vi "air formulas (SubVI).vi"(6 "Airflow Offset":dbl, 9 "Air Pressure Offset":dbl, 10 "Numeric in":u16, 11 "Numeric 4":u16) -> (2 "Numeric out":dbl, 3 "Numeric 3":dbl)   [LabVIEW 2016]
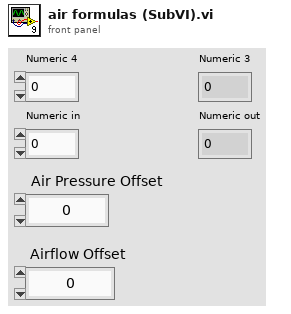
[diagram p1: front panel]
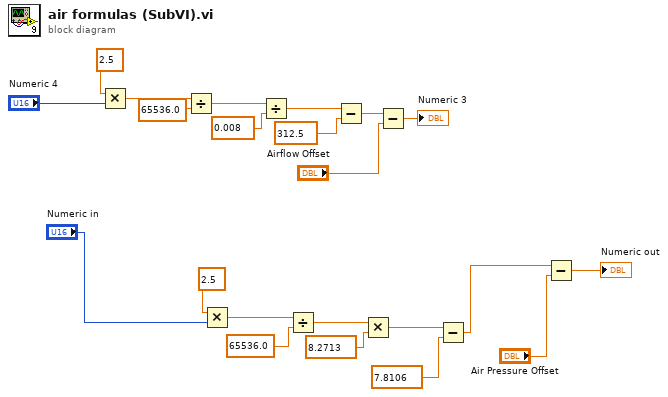
[diagram p0: block diagram]
diagram:
  n1 = Multiply(x=2.5, y="Numeric 4") -> (x*y=w12:dbl)
  n2 = Divide(x=w12, y=65536.0) -> (x/y=w14:dbl)
  n3 = Multiply(x=2.5, y="Numeric in") -> (x*y=w4:dbl)
  n4 = Divide(x=w14, y=0.008) -> (x/y=w16:dbl)
  n5 = Divide(x=w4, y=65536.0) -> (x/y=w6:dbl)
  n6 = Subtract(x=w16, y=312.5) -> (x-y=w18:dbl)
  n7 = Multiply(x=w6, y=8.2713) -> (x*y=w8:dbl)
  n8 = Subtract(x=w18, y="Airflow Offset") -> (x-y=→"Numeric 3":dbl)
  n9 = Subtract(x=w8, y=7.8106) -> (x-y=w2:dbl)
  n10 = Subtract(x=w2, y="Air Pressure Offset") -> (x-y=→"Numeric out":dbl)
